vi "TCP Data Read.vi"(8 "error in (no error)":errorcluster, 11 "Connection ID in":refnum<k5>) -> (0 "error out":errorcluster, 1 "Timeout error":bool, 2 "TCP Read data":string, 3 "Connection ID out":refnum<k5>)   [LabVIEW 2019, in "DeltaPSControl Shared.lvlib"]
uses:
  Shared/DeltaPSControl Shared.lvlib
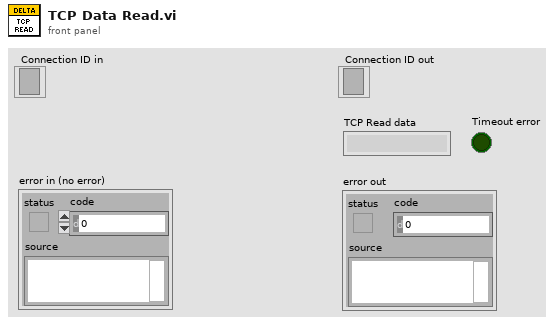
[diagram p1: front panel]
types:
  T1 = enum16{"Standard", "Buffered", "CRLF", "Immediate"}
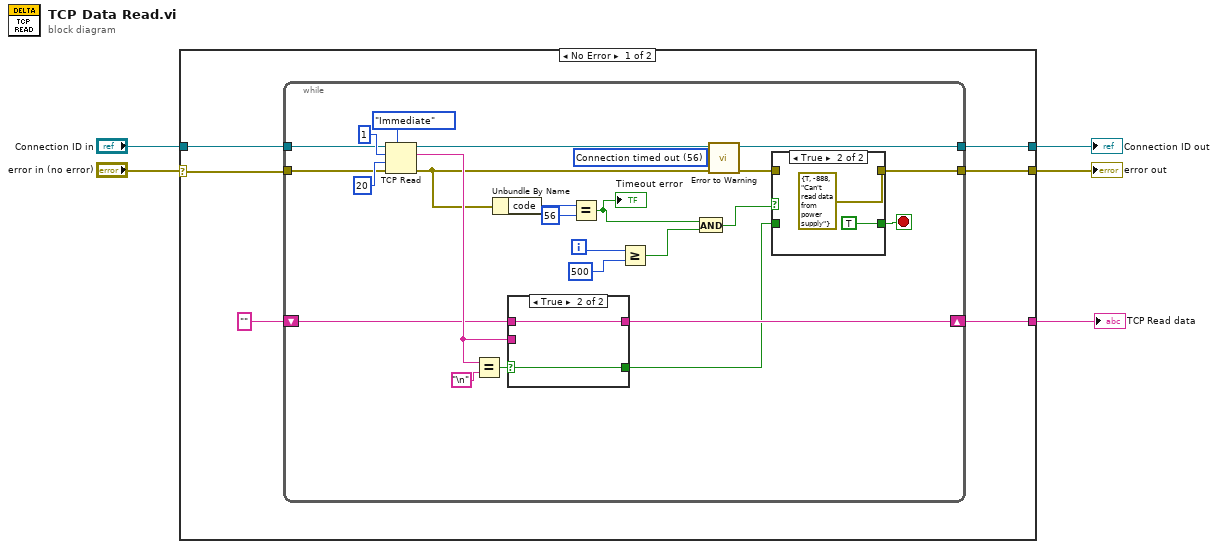
[diagram p0: block diagram]
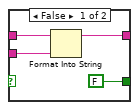
[diagram p3: hidden frame]
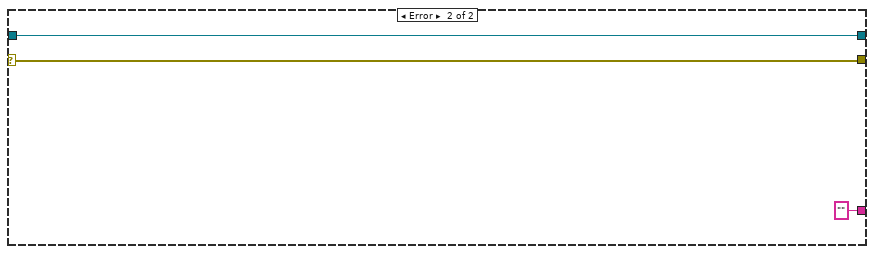
[diagram p4: hidden frame]
diagram:
  n1 = case shown="No Error" "error in (no error)" {
    selector: "error in (no error)" -> [w6 w48]
    tunnel: "Connection ID in" -> [w11 w47]
    tunnel: [w10 w48] -> w4
    tunnel: [w8 w47] -> w3
    tunnel: [w7 "" ("initial string")] -> w2
    frame No Error {
      n2 = while {
        tunnel: w6 -> [w33]
        tunnel: w11 -> [w32]
        tunnel: [w12] -> w10
        tunnel: [w31] -> w8
        shift-right: [w27] -> w7
        shift-left: "" ("initial string") -> [w28]
        i -> [w20]
        stop <- w16 stop-if-true
        w25 = 56 items=["No Error", "Argument Error", "Memory Full", "Out of Zone", "End of File", "File Already Open", "Generic File IO Error", "File Not Found", "File Permission Error", "Disk Full", "Duplicate Path", "Too Many Files Open", "Not Enabled", "Resource File Not Found", "Cannot Add Resource", "Resource Not Found", "Image Not Found", "Image Memory Error", "Pen Does Not Exist", "Config Bad Type", "Config Token Not Found", "Config Parse Error", "Config Memory Error", "Bad External Code Format", "Bad External Code Offset", "External Code Not Present", "Null Window", "Destroy Window Mixup", "Null Menu", "Print Aborted", "Bad Print Record", "Print Driver Error", "Windows Error During Print", "Memory Error During Print", "Print Dialog Error", "Generic Print Error", "Invalid Device Refnum", "Device Not Found", "Device Parameter Error", "Device Unit Error", "Can't Open Device", "Device Call Aborted", "Generic Error", "Cancelled By User", "Object ID Too Low", "Object ID Too High", "Object Not In Heap", "Unknown Heap", "Bad DefProc ID", "DefProc Not In Table", "Message Out Of Range", "Null Method", "Unknown Message", "Manager Call Not Supported", "Bad address", "Connection In progress", "Connection timed out", "Connection is already in progress", "Network attribute not supported", "Network error", "Address in use", "System out of memory", "Connection aborted", "Connection refused", "Connection is not connected", "Connection is already connected", "Connection closed", "Initialize error (interapplication manager)", "Bad occurrence", "Wait on unbound occurrence handler", "Occurrence queue overflow", "Bad path", "Semaphore not signaled", "Unrecognized type (interapplication manager)"] ("1st Error to Convert")
        n3 = TCP Read(connection ID=w32, bytes to read=1, error in (no error)=w33, 7:T1."Immediate" ("mode (standard)"), 9:20 ("timeout ms (25000)")) -> (connection ID out=w31:refnum<k5>, data out=w29:string, error out=w24:errorcluster)
        n4 = Equal?(x=w29, y="\n") -> (x = y?=w26:bool)
        n5 = Unbundle By Name(w24) -> ("code"=w22:i32)
        n6 = case shown="True" w26 {
          selector: w26 -> [_ w45]
          tunnel: w29 -> [w43 _]
          tunnel: w28 -> [w42 w44]
          tunnel: [w41 w44] -> w27
          tunnel: [FALSE w45] -> w18
          frame False {
            n7 = Format Into String(initial string=w42, w43) -> (resulting string=w41:string)  [unwired: 2 in, 1 out]
          }
          frame True {
          }
        }
        n8 = Equal?(x=w22, y=56) -> (x = y?=w15:bool)
        "Timeout error" <- w15
        n9 = Greater Or Equal?(x=w20, y=500) -> (x >= y?=w14:bool)
        n10 = And(x=w15, y=w14) -> (x .and. y?=w17:bool)
        n11 = call <vilib>:"Error to Warning.vi"("1st Error to Convert"=w25, "error in"=w24) -> ("warning out"=w13:errorcluster)  [unwired: 13 in]
        n12 = case shown="True" w17 {
          tunnel: w18 -> [w37 _]
          tunnel: [w37 TRUE] -> w16
          tunnel: w13 -> [w36 _]
          tunnel: [w36 errorcluster {"status"=TRUE, "code"=-888, "source"="Can't read data from power supply"} ("warning out")] -> w12
          frame False {
          }
          frame True {
          }
        }
      }
    }
    frame Error {
    }
  }
  "error out" <- w4
  "Connection ID out" <- w3
  "TCP Read data" <- w2
